vi "Coord window-Unbundle exp params.vi"(11 "Item Names + exp params":string[][](array[string])=[["PARAMETERS", "", "", ""], ["Zoom", "1", "", ""], ["FOV", "175", "", ""], ["", "", "", ""], ["COORDINATES & INFO", "", "", ""], ["2342", "67", "efge", ""], ["2354", "235", "drfg", ""], ["34", "3", "dge", ""], ["22", "33", "", "dh"], ["11", "56", "dg", ""]]) -> (3 "Item Names":string[][](array[string]))   [LabVIEW 2020]
uses:
  Globals/Coord window-Globals.vi
panel:
  out "Column names":string[](array[string])
  out "Parameters strings array":string[][](array[string])
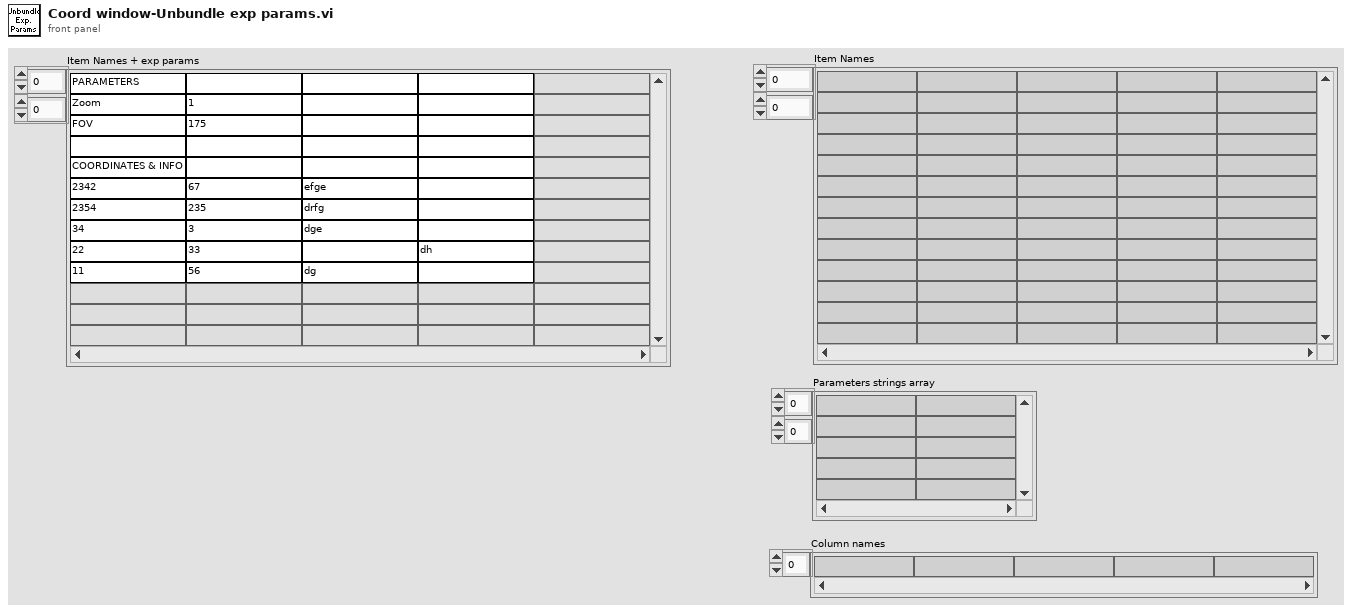
[diagram p1: front panel]
types:
  T1 = typedef "Coordinate list window refs.ctl" = cluster{"Window Name (i.e. Key)":string, "menu reference":refnum<k9>, "VI's reference":refnum<vi>, "Pane 1":refnum<vi>, "Pane 2":refnum<vi>, "Coord Listbox":refnum<vi>, "File name":refnum<vi>, "Picture Map":refnum<vi>, "Stage XYZ Position ind.":refnum<vi>}
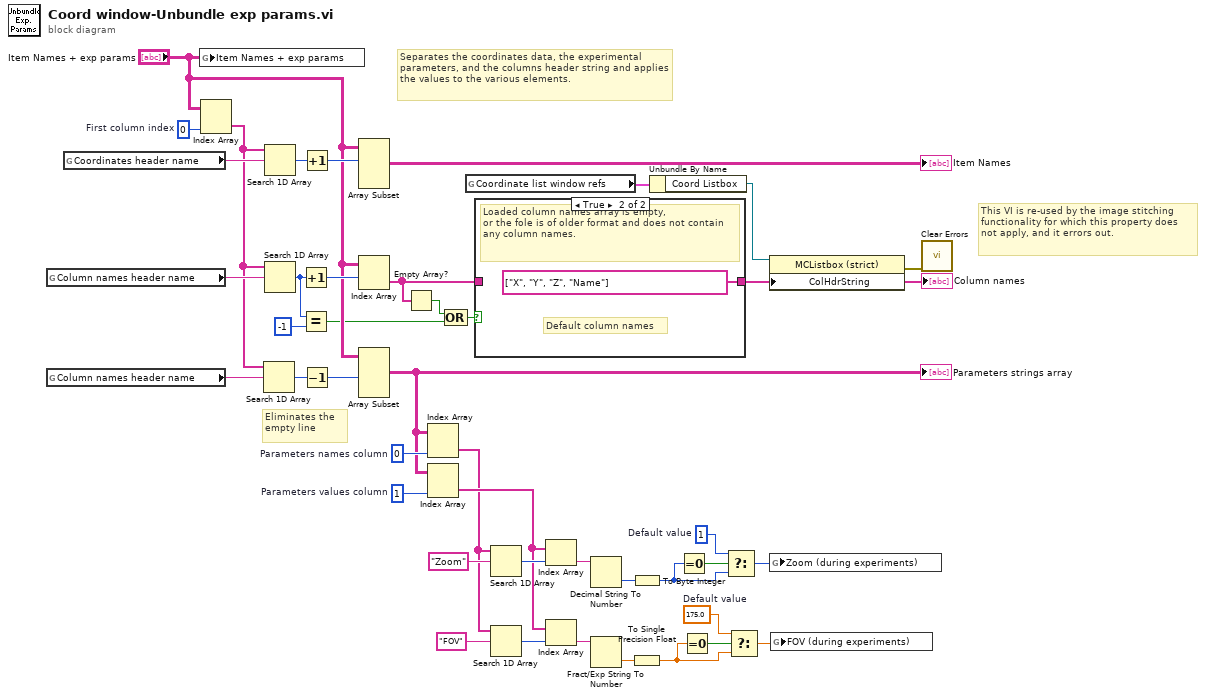
[diagram p0: block diagram]
diagram:
  w14 = 0  # First column index
  w26 = sgl 175.0  # Default value
  w27 = i8 1  # Default value
  w39 = 1  # Parameters values column
  w41 = 0  # Parameters names column
  # "This VI is re-used by the image stitching functionality for which this property does not apply, and it errors out."
  # "Separates the coordinates data, the experimental parameters, and the columns header string and applies the values to the various elements."
  # "Eliminates the empty line"
  n1 = global read "Coord window-Globals.vi" "Column names header name"() -> (w15:string)
  n2 = global read "Coord window-Globals.vi" "Column names header name"() -> (w19:string)
  n3 = global read "Coord window-Globals.vi" "Coordinates header name"() -> (w20:string)
  n4 = global write "Coord window-Globals.vi" "Item Names + exp params"("Item Names + exp params") -> ()
  n5 = Index Array(array="Item Names + exp params", index (col)=w14) -> (element=w13:string[])  [unwired: 1 in]
  n6 = Search 1D Array(1D array=w13, element=w19) -> (index of element=w22:i32)  [unwired: 1 in]
  n7 = Search 1D Array(1D array=w13, element=w20) -> (index of element=w21:i32)  [unwired: 1 in]
  n8 = Search 1D Array(1D array=w13, element=w15) -> (index of element=w6:i32)  [unwired: 1 in]
  n9 = Increment(x=w6) -> (x+1=w17:i32)
  n10 = Equal?(x=w6, y=-1) -> (x = y?=w4:bool)
  n11 = Increment(x=w21) -> (x+1=w43:i32)
  n12 = Decrement(x=w22) -> (x-1=w42:i32)
  n13 = Array Subset(array="Item Names + exp params", index (row)=w43) -> (→"Item Names":string[][])  [unwired: 3 in]
  n14 = Index Array(array="Item Names + exp params", index (row)=w17) -> (element=w9:string[])  [unwired: 1 in]
  n15 = Array Subset(array="Item Names + exp params", length (row)=w42) -> (w10:string[][])  [unwired: 3 in]
  "Parameters strings array" <- w10
  n16 = Empty Array?(array=w9) -> (empty?=w3:bool)
  n17 = Index Array(array=w10, index (col)=w41) -> (element=w18:string[])  [unwired: 1 in]
  n18 = Index Array(array=w10, index (col)=w39) -> (element=w36:string[])  [unwired: 1 in]
  n19 = Compound Arithmetic op=OR(w3, w4) -> (w2:bool)
  n20 = global read "Coord window-Globals.vi" "Coordinate list window refs"() -> (w12:T1)
  n21 = case shown="True" w2 {
    tunnel: w9 -> [w44 _]
    tunnel: [w44 string[] ["X", "Y", "Z", "Name"] ("Column names")] -> w8
    frame False {
    }
    frame True {
      # "Default column names"
      # "Loaded column names array is empty,\nor the fole is of older format and does not contain any column names."
    }
  }
  "Column names" <- w8
  n22 = Search 1D Array(1D array=w18, element="Zoom") -> (index of element=w37:i32)  [unwired: 1 in]
  n23 = Search 1D Array(1D array=w18, element="FOV") -> (index of element=w35:i32)  [unwired: 1 in]
  n24 = Index Array(array=w36, index=w37) -> (element=w34:string)
  n25 = Index Array(array=w36, index=w35) -> (element=w32:string)
  n26 = Decimal String To Number(string=w34) -> (number=w33:i32)  [unwired: 2 in, 1 out]
  n27 = Fract/Exp String To Number(string=w32) -> (number=w31:dbl)  [unwired: 3 in, 1 out]
  n28 = To Byte Integer(number=w33) -> (8bit integer=w28:i8)
  n29 = To Single Precision Float(number=w31) -> (single precision float=w24:sgl)
  n30 = Unbundle By Name(w12) -> ("Coord Listbox"=w11:refnum<vi>)
  n31 = Equal To 0?(x=w28) -> (x = 0?=w30:bool)
  n32 = Equal To 0?(x=w24) -> (x = 0?=w25:bool)
  n33 = Select(t=w27, s=w30, f=w28) -> (s? t:f=w29:i8)
  n34 = Select(t=w26, s=w25, f=w24) -> (s? t:f=w23:sgl)
  n35 = property on="Property Node" class="MCListbox (strict)"(reference=w11, "ColHdrString"=w8) -> (error out=w1:errorcluster)  [unwired: 1 in, 1 out]
  n36 = global write "Coord window-Globals.vi" "Zoom (during experiments)"(w29) -> ()
  n37 = global write "Coord window-Globals.vi" "FOV (during experiments)"(w23) -> ()
  n38 = call <vilib>:"Clear Errors.vi"("error in (no error)"=w1) -> ()  [unwired: 5 in, 2 out]
